vi "Remove Service.vi"(8 "error in (no error)":errorcluster, 10 "Service":refnum<class "Service.lvclass">, 11 "Service Container in":refnum<class "Service Container.lvclass">) -> (0 "error out":errorcluster, 3 "Service Container out":refnum<class "Service Container.lvclass">)   [LabVIEW 2020, in "Vecto.lvlib" / "Service Container.lvclass"]
uses:
  Service Container.lvclass
  Service/Service.lvclass
  Service Container.lvclass/Service Container.ctl
  <vilib>/Utility/miscctls.llb/LVMapReplaceAction.ctl
  <vilib>/Utility/error.llb/Error Cluster From Error Code.vi
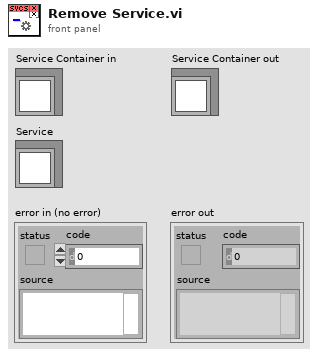
[diagram p1: front panel]
types:
  T1 = typedef "LVMapReplaceAction.ctl" = enum32{"Modify Entry only if found", "Add or Modify Entry", "Delete Entry"}
  T2 = typedef "Vecto.lvlib/Service Container.lvclass/Services.ctl" = map{string, map{string, refnum<class "Service.lvclass">}}
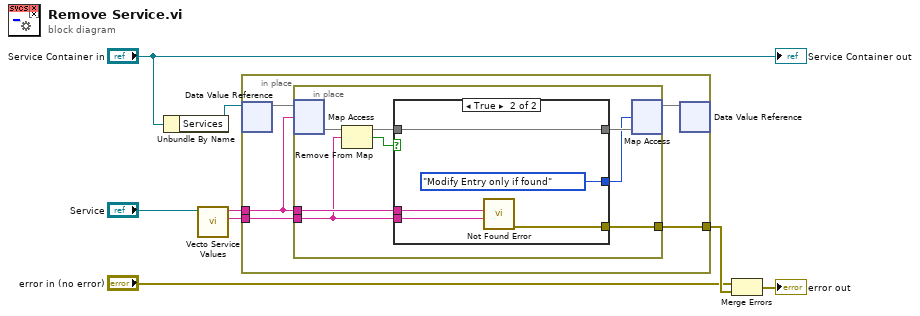
[diagram p0: block diagram]
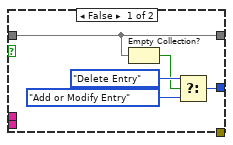
[diagram p2: hidden frame]
diagram:
  n1 = Unbundle By Name("Service Container in") -> ("Services"=w7:refnum<data-value>)
  n2 = call "Vecto Service Values.vi"("Service in"="Service") -> ("ID"=w5:string, "Type"=w6:string)  [unwired: 9 in]
  n3 = in-place {
    in-place-border: w6 -> [w10]
    in-place-border: w5 -> [w12]
    in-place-border: [w9] -> w3
    n4 = in-place-dvr #1(w7) -> (w13:T2)  [unwired: 1 out]
    n5 = in-place {
      in-place-border: w12 -> [w18]
      in-place-border: w10 -> [w21]
      in-place-border: [w20] -> w9
      n6 = in-place-map #2(w13, w10) -> (w19:map{string, refnum<class "Service.lvclass">})  [unwired: 1 in, 1 out]
      n7 = Remove From Map(10:w18, 11:w19) -> (2:w17:bool, 3:w16:map{string, refnum<class "Service.lvclass">})  [unwired: 1 out]
      n8 = case shown="True" w17 {
        tunnel: w18 -> [_ w28]
        tunnel: w21 -> [_ w29]
        tunnel: [_ w27] -> w20
        tunnel: w16 -> [w26 w30]
        tunnel: [w26 w30] -> w15
        tunnel: [w22 LVMapReplaceAction."Modify Entry only if found" ("action")] -> w14
        frame False {
          n9 = Empty Collection?(1:w26) -> (0:w23:bool)
          n10 = Select(t=LVMapReplaceAction."Delete Entry" ("action"), s=w23, f=LVMapReplaceAction."Add or Modify Entry" ("action")) -> (s? t:f=w22:T1)
        }
        frame True {
          n11 = call "Not Found Error.vi"("ID"=w28, "Type"=w29) -> ("error out"=w27:errorcluster)  [unwired: 9 in]
        }
      }
      n12 = in-place-map #2(w15, w14) -> (w11:T2)  [unwired: 2 out]
    }
    n13 = in-place-dvr #1(w11) -> ()  [unwired: 2 out]
  }
  n14 = Merge Errors("error in (no error)", w3) -> (→"error out":errorcluster)
  "Service Container out" <- "Service Container in"
